vi "testFlushTelQueueFromDds.vi"(8 "error in (no error)":errorcluster) -> (0 "error out":errorcluster)   [LabVIEW 2018]
doc: "Test the flushTelQueue.vi with queueFromDds option."
uses:
  src/FactoryTcpServer/FactoryTcpServer.lvclass
  src/TcpServer/TcpServer.lvclass/TcpServer.ctl
  src/TcpServerTel/TcpServerTel.lvclass/TcpServerTel.ctl
  src/TcpServerTel/TcpServerTel.lvclass
  home/pcortes/Documents/github/ts_labview_tcp_json/src/TcpServerBase/TcpServerBase.lvclass
  <vilib>/addons/_JKI Toolkits/Caraya/classes/Assert/Assert Equal Value_Variant.vi
  <vilib>/addons/_JKI Toolkits/Caraya/classes/Test/Test.lvclass
  <vilib>/addons/_JKI Toolkits/Caraya/classes/Assert/Assert.lvclass
  src/TcpServer/TcpServer.lvclass
  src/TcpServerBase/TcpServerBase.lvclass
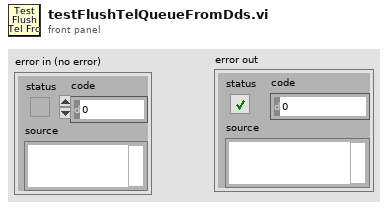
[diagram p1: front panel]
types:
  T1 = enum16{"queueTcpClientFromDds", "queueTcpClient"}
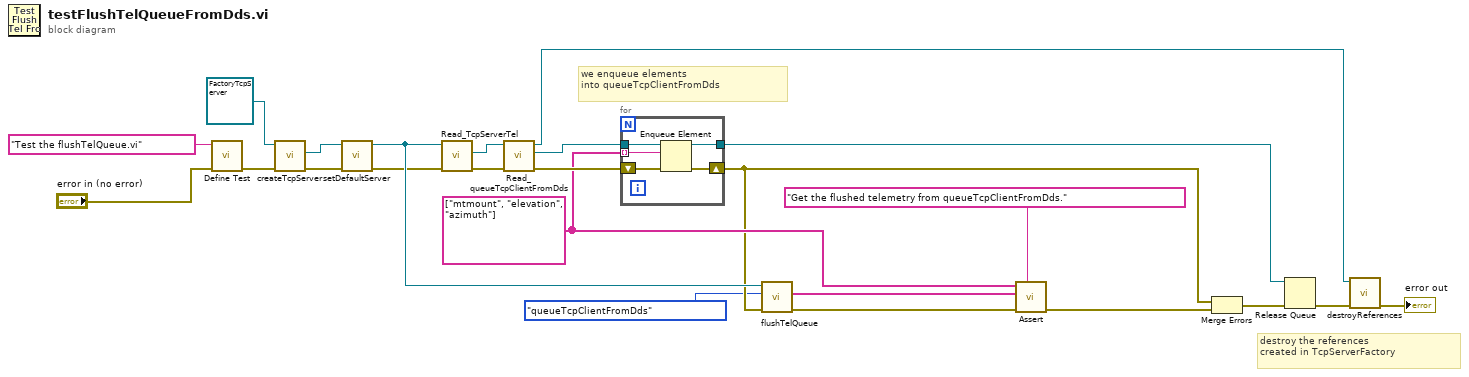
[diagram p0: block diagram]
diagram:
  w10 = string[] ["mtmount", "elevation", "azimuth"]
  # "destroy the references\ncreated in TcpServerFactory"
  # "we enqueue elements\ninto queueTcpClientFromDds"
  n1 = call <vilib>:"Define Test.vi"("error in (no error)"="error in (no error)", "Label (VI Title)"="Test the flushTelQueue.vi") -> ("error out"=w5:errorcluster)  [unwired: 9 in]
  n2 = call "createTcpServer.vi"("error in (no error)"=w5, "FactoryTcpServer in"=refnum<class "FactoryTcpServer.lvclass"> refnum) -> ("error out"=w4:errorcluster, "TcpServer out"=w6:refnum<class "TcpServer.lvclass">)  [unwired: 7 in, 1 out]
  n3 = call "setDefaultServer.vi"("error in (no error)"=w4, "TcpServer.lvclass"=w6) -> ("error out"=w13:errorcluster, "tcpServer out"=w14:refnum<class "TcpServer.lvclass">)  [unwired: 8 in]
  n4 = call "Read_TcpServerTel.vi"("error in (no error)"=w13, "TcpServer in"=w14) -> ("error out"=w19:errorcluster, "TcpServerTel.lvclass"=w20:refnum<class "TcpServerTel.lvclass">)  [unwired: 7 in, 1 out]
  n5 = call "Read_queueTcpClientFromDds.vi"("error in (no error)"=w19, "TcpServerTel in"=w20) -> ("error out"=w17:errorcluster, "queueTcpClientFromDds"=w16:refnum<queue>, "TcpServerTel out"=w1:refnum<class "TcpServerTel.lvclass">)  [unwired: 7 in]
  n6 = for {
    tunnel: w16 -> [w28]
    tunnel: w10 -> [w27] mode=indexing
    tunnel: [w25] -> w15
    shift-right: [w26] -> w9
    shift-left: w17 -> [w29]
    n7 = Enqueue Element(queue=w28, element=w27, error in (no error)=w29) -> (queue out=w25:refnum<queue>, error out=w26:errorcluster)  [unwired: 1 in, 1 out]
  }
  n8 = call "flushTelQueue.vi"("error in (no error)"=w9, "queueName"=T1."queueTcpClientFromDds", "TcpServer in"=w14) -> ("error out"=w12:errorcluster, "telemetry flushed"=w11:string[])  [unwired: 6 in, 1 out]
  n9 = call-poly <vilib>:"Assert.vi"("Label"="Get the flushed telemetry from queueTcpClientFromDds.", "error in (no error)"=w12, "Y"=w11, "X"=w10) -> ("error out"=w21:errorcluster)  [unwired: 7 in]
  n10 = Merge Errors(w9, w21) -> (w18:errorcluster)
  n11 = Release Queue(queue=w15, error in (no error)=w18) -> (error out=w3:errorcluster)  [unwired: 1 in, 2 out]
  n12 = call "destroyReferences.vi"("error in (no error)"=w3, "tcpServerBase in"=w1) -> ("error out"=→"error out":errorcluster)  [unwired: 8 in, 1 out]
